vi "GT Add Var Calculate.vi"(8 "error in (no error)":errorcluster caption="错误输入（无错误）", 9 "pIndex":i16, 10 "pVarCalculate":T1, 11 "cardNum":i16) -> (0 "error out":errorcluster caption="错误输出", 1 "pIndex out":i16, 2 "pVarCalculate out":T1, 3 "function return":i16)   [LabVIEW 2020, in "gts1.lvlib"]
doc: "GT_API GT_AddVarCalculate(short cardNum,TVarCalculate *pVarCalculate,short *pIndex);"
uses:
  gts1.lvlib
  dll/32bit/multi_card/gts.dll
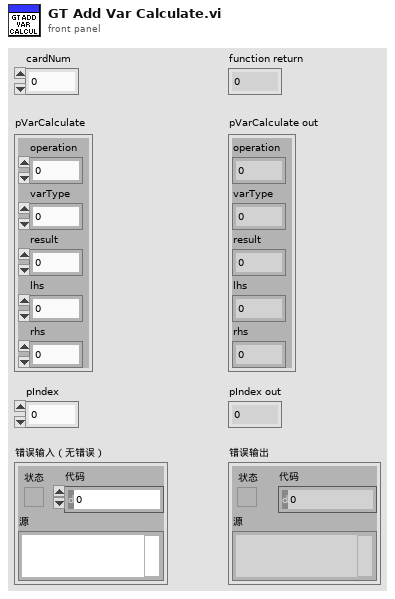
[diagram p1: front panel]
types:
  T1 = cluster{"operation":u16, "varType":u16, "result":u16, "lhs":u16, "rhs":u16}
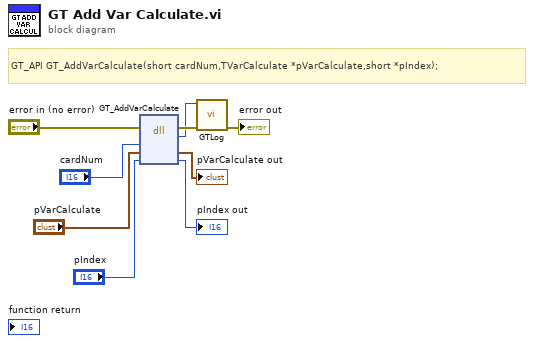
[diagram p0: block diagram]
diagram:
  # "GT_API GT_AddVarCalculate(short cardNum,TVarCalculate *pVarCalculate,short *pIndex);"
  n1 = dll-call lib="C:/1228/dll/32bit/multi_card/gts.dll" fn="GT_AddVarCalculate"(error in="error in (no error)", "cardNum"="cardNum", "pVarCalculate"="pVarCalculate", "pIndex"="pIndex") -> (error out=w3:errorcluster, w1:i16, "pVarCalculate"=→"pVarCalculate out":T1, "pIndex"=→"pIndex out":i16)  [unwired: 3 in, 1 out]
  n2 = call "GTLog.vi"("error in (no error)"=w3, "Numeric"=w1) -> ("error out"=→"error out":errorcluster)  [unwired: 9 in]
